vi "Offset Inline Buffer.vi"(8 "error in (no error)":errorcluster, 10 "base Inline Buffer":refnum<class "Buffer.lvclass">, 11 "Buffers in":refnum<class "Buffers.lvclass">) -> (0 "error out":errorcluster, 3 "Buffers out":refnum<class "Buffers.lvclass">)   [LabVIEW 2017, in "DSF Core.lvlib" / "Buffers.lvclass"]
uses:
  Buffers.lvclass
  Buffer/Buffer.lvclass
  Buffers.lvclass/Buffers.ctl
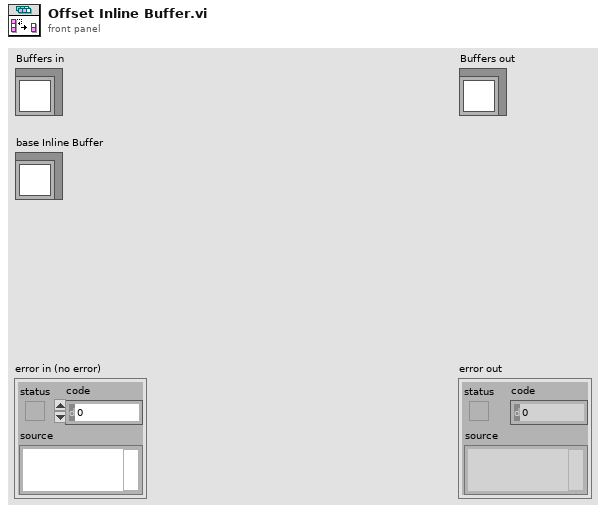
[diagram p1: front panel]
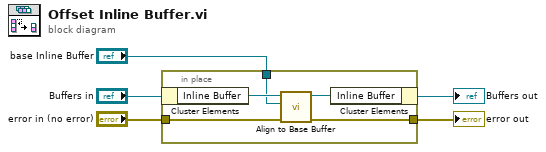
[diagram p0: block diagram]
diagram:
  n1 = in-place {
    in-place-border: "error in (no error)" -> [w8]
    in-place-border: [w7] -> w3
    in-place-border: "base Inline Buffer" -> [w6]
    n2 = in-place-cluster #1("Buffers in") -> ("Inline Buffer"=w10:refnum<class "Buffer.lvclass">)
    n3 = call "Align to Base Buffer.vi"("error in (no error)"=w8, "base Buffer"=w6, "Buffer in"=w10) -> ("error out"=w7:errorcluster, "Buffer out"=w9:refnum<class "Buffer.lvclass">)  [unwired: 7 in]
    n4 = in-place-cluster #1("Inline Buffer"=w9) -> (→"Buffers out":refnum<class "Buffers.lvclass">)
  }
  "error out" <- w3
